vi "LOC subReplaceNewLineCharWithHexChar0x0A.vi"(1 "InputString":string) -> (0 "OutputString":string)   [LabVIEW 2020, in "Localization_Tools.lvlib"]
uses:
  Localization_Tools.lvlib
panel:
  # "Because some control labels/captions/etc can have '\\n' newline characters\nin them, we must flatten these to work with INI file format.  This VI will replace\nall \\n chars with \\0A, which is then interpreted by the INI/XML converters\nas <LF/>"
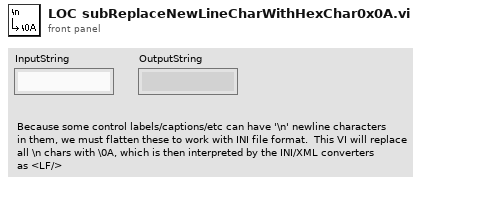
[diagram p1: front panel]
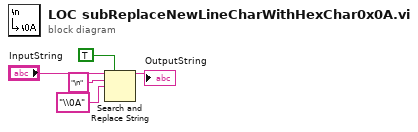
[diagram p0: block diagram]
diagram:
  n1 = Search and Replace String(replace all?=TRUE ("replace all? (F)"), input string="InputString", search string="\n", replace string="\\0A" ("replace string (\"\")")) -> (result string=→"OutputString":string)  [unwired: 4 in, 3 out]
